vi "Read Settings FGV.vi"(6 "Option":enum16{"Read Settings", "Write Settings"}(ring), 8 "error in":errorcluster, 11 "Application Settings":T4) -> (0 "error out":errorcluster, 3 "Application Settings":T4)   [LabVIEW 2022 SP3, in "Controller.lvlib" / "Controller.lvclass"]
uses:
  Controller.lvclass
  <vilib>/Utility/config.llb/NI_LVConfig.lvlib
  <vilib>/Utility/config.llb/Read Key (U32).vi
  <vilib>/Utility/config.llb/Read Key (Path).vi
  <vilib>/Utility/config.llb/Read Key (Boolean).vi
  <vilib>/Utility/config.llb/Read Key (String).vi
  <vilib>/Utility/config.llb/Write Key (Boolean).vi
  <vilib>/Utility/config.llb/Write Key (Path).vi
  <vilib>/Utility/config.llb/Write Key (String).vi
  <vilib>/Utility/config.llb/Write Key (U32).vi
  Typedefs/PLC Settings.ctl
  Typedefs/Image Formats.ctl
  Typedefs/Storage Settings.ctl
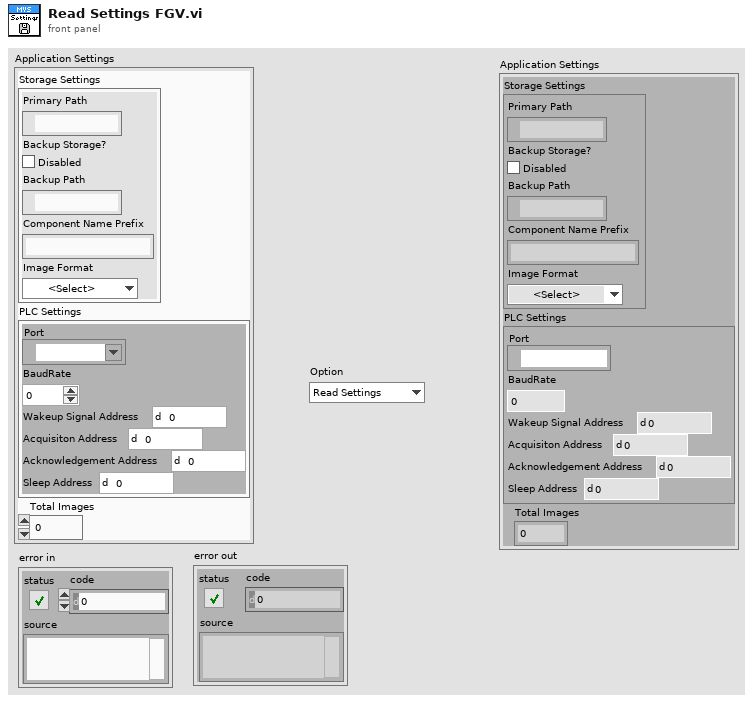
[diagram p1: front panel]
types:
  T1 = typedef "Storage Settings.ctl" = cluster{"Primary Path":path, "Backup Storage?":bool, "Backup Path":path, "Component Name Prefix":string, "Image Format":T2}
  T2 = typedef "Image Formats.ctl" = enum16{"<Select>", "TIFF", "RAW"}
  T3 = typedef "PLC Settings.ctl" = cluster{"Port":refnum<visa-resource-name>, "BaudRate":u32, "Wakeup Signal Address ":u16, "Acquisiton Address":u16, "Acknowledgement Address":u16, "Sleep Address":u16}
  T4 = cluster{"Storage Settings":T1, "PLC Settings":T3, "Total Images":u32}
  T5 = typedef "NI_LVConfig.lvlib/Config Data RefNum.ctl" = refnum<k1>
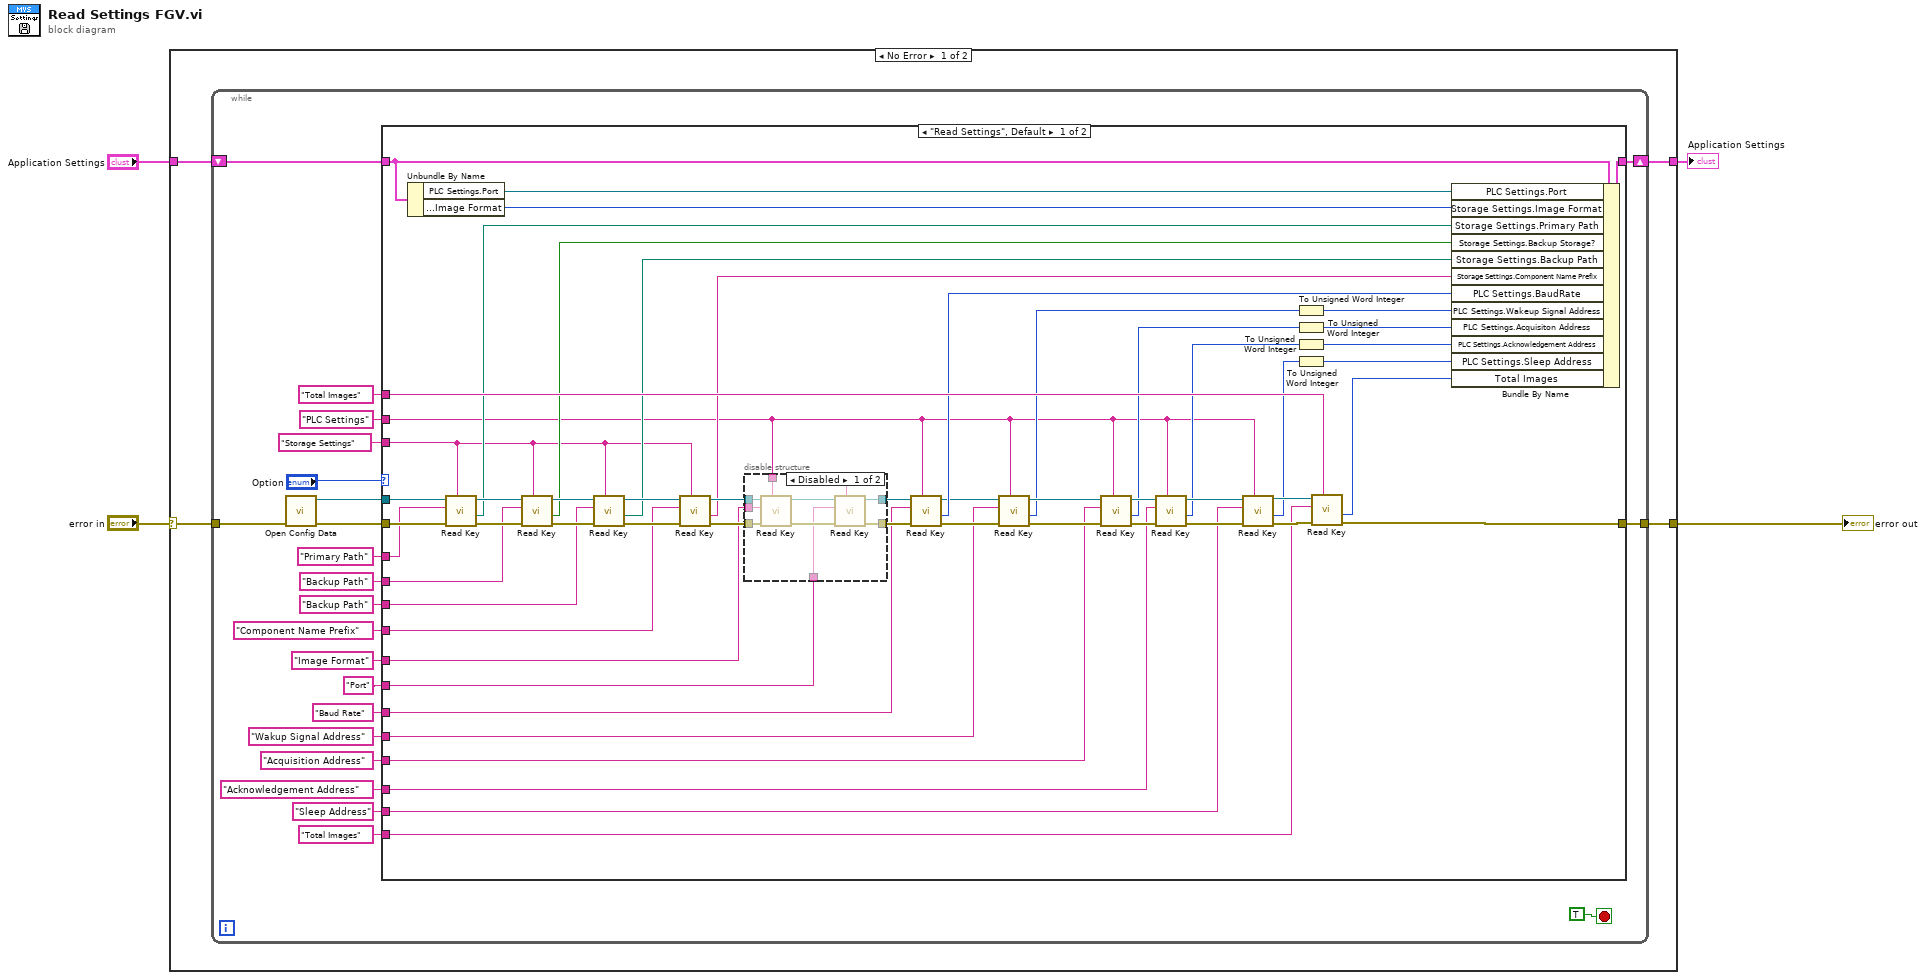
[diagram p0: block diagram]
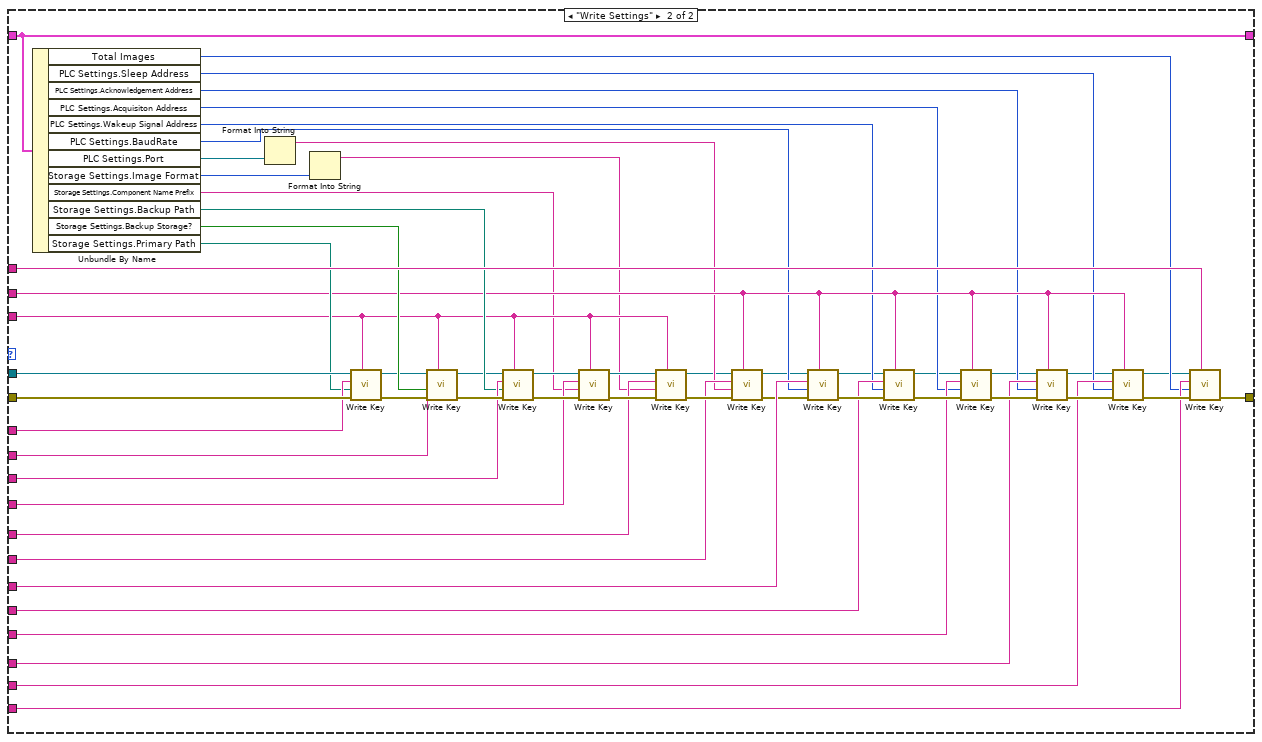
[diagram p3: hidden frame]
diagram:
  n1 = case shown="No Error" "error in" {
    selector: "error in" -> [w8 w155]
    tunnel: [w7 w155] -> w3
    tunnel: "Application Settings" -> [w6 w154]
    tunnel: [w5 w154] -> w1
    frame No Error {
      n2 = while {
        tunnel: w8 -> [w30]
        tunnel: [w26] -> w7
        shift-right: [w21] -> w5
        shift-left: w6 -> [w25]
        stop <- TRUE stop-if-true
        n3 = call <vilib>:"Open Config Data.vi"("error in (no error)"=w30) -> ("error out"=w28:errorcluster, "refnum"=w27:T5)  [unwired: 8 in, 1 out]
        n4 = case shown="\"Read Settings\", Default" "Option" {
          tunnel: w28 -> [w87 w153]
          tunnel: w27 -> [w67 w132]
          tunnel: [w78 w144] -> w26
          tunnel: w25 -> [w34 w133]
          tunnel: "PLC Settings" -> [w37 w119]
          tunnel: "Storage Settings" -> [w38 w121]
          tunnel: "Total Images" -> [w75 w140]
          tunnel: [w74 w133] -> w21
          tunnel: "Primary Path" -> [w48 w143]
          tunnel: "Backup Path" -> [w47 w142]
          tunnel: "Backup Path" -> [w46 w141]
          tunnel: "Component Name Prefix" -> [w45 w116]
          tunnel: "Baud Rate" -> [w39 w134]
          tunnel: "Wakup Signal Address" -> [w44 w135]
          tunnel: "Acquisition Address" -> [w43 w136]
          tunnel: "Acknowledgement Address" -> [w42 w137]
          tunnel: "Sleep Address" -> [w41 w138]
          tunnel: "Total Images" -> [w40 w139]
          tunnel: "Image Format" -> [w35 w124]
          tunnel: "Port" -> [w36 w120]
          frame "Read Settings", Default {
            n5 = Unbundle By Name(w34) -> ("PLC Settings.Port"=w32:refnum<visa-resource-name>, "Storage Settings.Image Format"=w33:T2)
            n6 = call-poly <vilib>:"Read Key.vi"("section"=w38, "error in (no error)"=w87, "key"=w48, "refnum"=w67) -> ("error out"=w76:errorcluster, "value"=w60:path, "refnum out"=w66:T5)  [unwired: 4 in, 1 out]
            n7 = call-poly <vilib>:"Read Key.vi"("section"=w38, "error in (no error)"=w76, "key"=w47, "refnum"=w66) -> ("error out"=w86:errorcluster, "value"=w59:bool, "refnum out"=w65:T5)  [unwired: 4 in, 1 out]
            n8 = call-poly <vilib>:"Read Key.vi"("section"=w38, "error in (no error)"=w86, "key"=w46, "refnum"=w65) -> ("error out"=w85:errorcluster, "value"=w58:path, "refnum out"=w64:T5)  [unwired: 4 in, 1 out]
            n9 = call-poly <vilib>:"Read Key.vi"("section"=w38, "error in (no error)"=w85, "key"=w45, "refnum"=w64) -> ("error out"=w84:errorcluster, "value"=w57:string, "refnum out"=w63:T5)  [unwired: 4 in, 1 out]
            n10 = disable-structure shown="Disabled" {
              disable-tunnel: w84 -> [w96 w98]
              disable-tunnel: [w95 w98] -> w77
              disable-tunnel: w37 -> [w93 _]
              disable-tunnel: w63 -> [w92 w97]
              disable-tunnel: [w90 w97] -> w62
              disable-tunnel: w35 -> [w89 _]
              disable-tunnel: w36 -> [w88 _]
              frame Disabled {
                n11 = call-poly <vilib>:"Read Key.vi"("section"=w93, "error in (no error)"=w96, "key"=w89, "refnum"=w92) -> ("error out"=w94:errorcluster, "refnum out"=w91:T5)  [unwired: 4 in, 2 out]
                n12 = call-poly <vilib>:"Read Key.vi"("section"=w93, "error in (no error)"=w94, "key"=w88, "refnum"=w91) -> ("error out"=w95:errorcluster, "refnum out"=w90:T5)  [unwired: 4 in, 2 out]
              }
              frame Enabled {
              }
            }
            n13 = call-poly <vilib>:"Read Key.vi"("section"=w37, "error in (no error)"=w77, "key"=w39, "refnum"=w62) -> ("error out"=w83:errorcluster, "value"=w73:u32, "refnum out"=w61:T5)  [unwired: 4 in, 1 out]
            n14 = call-poly <vilib>:"Read Key.vi"("section"=w37, "error in (no error)"=w83, "key"=w44, "refnum"=w61) -> ("error out"=w82:errorcluster, "value"=w54:u32, "refnum out"=w68:T5)  [unwired: 4 in, 1 out]
            n15 = call-poly <vilib>:"Read Key.vi"("section"=w37, "error in (no error)"=w82, "key"=w43, "refnum"=w68) -> ("error out"=w81:errorcluster, "value"=w52:u32, "refnum out"=w69:T5)  [unwired: 4 in, 1 out]
            n16 = call-poly <vilib>:"Read Key.vi"("section"=w37, "error in (no error)"=w81, "key"=w42, "refnum"=w69) -> ("error out"=w80:errorcluster, "value"=w56:u32, "refnum out"=w70:T5)  [unwired: 4 in, 1 out]
            n17 = call-poly <vilib>:"Read Key.vi"("section"=w37, "error in (no error)"=w80, "key"=w41, "refnum"=w70) -> ("error out"=w79:errorcluster, "value"=w55:u32, "refnum out"=w71:T5)  [unwired: 4 in, 1 out]
            n18 = To Unsigned Word Integer(number=w54) -> (unsigned 16bit integer=w53:u16)
            n19 = To Unsigned Word Integer(number=w52) -> (unsigned 16bit integer=w51:u16)
            n20 = To Unsigned Word Integer(number=w56) -> (unsigned 16bit integer=w50:u16)
            n21 = To Unsigned Word Integer(number=w55) -> (unsigned 16bit integer=w49:u16)
            n22 = call-poly <vilib>:"Read Key.vi"("section"=w75, "error in (no error)"=w79, "key"=w40, "refnum"=w71) -> ("error out"=w78:errorcluster, "value"=w72:u32)  [unwired: 4 in, 2 out]
            n23 = Bundle By Name(cluster=w34, "PLC Settings.Port"=w32, "Storage Settings.Image Format"=w33, "Storage Settings.Primary Path"=w60, "Storage Settings.Backup Storage?"=w59, "Storage Settings.Backup Path"=w58, "Storage Settings.Component Name Prefix"=w57, "PLC Settings.BaudRate"=w73, "PLC Settings.Wakeup Signal Address"=w53, "PLC Settings.Acquisiton Address"=w51, "PLC Settings.Acknowledgement Address"=w50, "PLC Settings.Sleep Address"=w49, "Total Images"=w72) -> (w74:T4)
          }
          frame "Write Settings" {
            n24 = Unbundle By Name(w133) -> ("Total Images"=w107:u32, "PLC Settings.Sleep Address"=w106:u16, "PLC Settings.Acknowledgement Address"=w108:u16, "PLC Settings.Acquisiton Address"=w109:u16, "PLC Settings.Wakeup Signal Address"=w110:u16, "PLC Settings.BaudRate"=w111:u32, "PLC Settings.Port"=w117:refnum<visa-resource-name>, "Storage Settings.Image Format"=w118:T2, "Storage Settings.Component Name Prefix"=w115:string, "Storage Settings.Backup Path"=w129:path, "Storage Settings.Backup Storage?"=w130:bool, "Storage Settings.Primary Path"=w131:path)
            n25 = Format Into String(w117) -> (resulting string=w113:string)  [unwired: 3 in, 1 out]
            n26 = Format Into String(w118) -> (resulting string=w114:string)  [unwired: 3 in, 1 out]
            n27 = call-poly <vilib>:"Write Key.vi"("section"=w121, "error in (no error)"=w153, "value"=w131, "key"=w143, "refnum"=w132) -> ("error out"=w148:errorcluster, "refnum out"=w128:T5)  [unwired: 4 in, 1 out]
            n28 = call-poly <vilib>:"Write Key.vi"("section"=w121, "error in (no error)"=w148, "value"=w130, "key"=w142, "refnum"=w128) -> ("error out"=w151:errorcluster, "refnum out"=w127:T5)  [unwired: 4 in, 1 out]
            n29 = call-poly <vilib>:"Write Key.vi"("section"=w121, "error in (no error)"=w151, "value"=w129, "key"=w141, "refnum"=w127) -> ("error out"=w147:errorcluster, "refnum out"=w123:T5)  [unwired: 4 in, 1 out]
            n30 = call-poly <vilib>:"Write Key.vi"("section"=w121, "error in (no error)"=w147, "value"=w115, "key"=w116, "refnum"=w123) -> ("error out"=w126:errorcluster, "refnum out"=w122:T5)  [unwired: 4 in, 1 out]
            n31 = call-poly <vilib>:"Write Key.vi"("section"=w121, "error in (no error)"=w126, "value"=w114, "key"=w124, "refnum"=w122) -> ("error out"=w125:errorcluster, "refnum out"=w105:T5)  [unwired: 4 in, 1 out]
            n32 = call-poly <vilib>:"Write Key.vi"("section"=w119, "error in (no error)"=w125, "value"=w113, "key"=w120, "refnum"=w105) -> ("error out"=w112:errorcluster, "refnum out"=w104:T5)  [unwired: 4 in, 1 out]
            n33 = call-poly <vilib>:"Write Key.vi"("section"=w119, "error in (no error)"=w112, "value"=w111, "key"=w134, "refnum"=w104) -> ("error out"=w150:errorcluster, "refnum out"=w103:T5)  [unwired: 4 in, 1 out]
            n34 = call-poly <vilib>:"Write Key.vi"("section"=w119, "error in (no error)"=w150, "value"=w110, "key"=w135, "refnum"=w103) -> ("error out"=w146:errorcluster, "refnum out"=w102:T5)  [unwired: 4 in, 1 out]
            n35 = call-poly <vilib>:"Write Key.vi"("section"=w119, "error in (no error)"=w146, "value"=w109, "key"=w136, "refnum"=w102) -> ("error out"=w152:errorcluster, "refnum out"=w101:T5)  [unwired: 4 in, 1 out]
            n36 = call-poly <vilib>:"Write Key.vi"("section"=w119, "error in (no error)"=w152, "value"=w108, "key"=w137, "refnum"=w101) -> ("error out"=w145:errorcluster, "refnum out"=w100:T5)  [unwired: 4 in, 1 out]
            n37 = call-poly <vilib>:"Write Key.vi"("section"=w119, "error in (no error)"=w145, "value"=w106, "key"=w138, "refnum"=w100) -> ("error out"=w149:errorcluster, "refnum out"=w99:T5)  [unwired: 4 in, 1 out]
            n38 = call-poly <vilib>:"Write Key.vi"("section"=w140, "error in (no error)"=w149, "value"=w107, "key"=w139, "refnum"=w99) -> ("error out"=w144:errorcluster)  [unwired: 4 in, 2 out]
          }
        }
      }
    }
    frame Error {
    }
  }
  "error out" <- w3
  "Application Settings" <- w1
